vi "GetObjectFromMemory.vi"(8 "error in (no error)":errorcluster, 10 "ObjectName":string, 11 "Type":refnum<class>) -> (0 "error out":errorcluster, 3 "ObjectOut":refnum<class>)   [LabVIEW 2021, in "Application.lvclass"]
uses:
  Application.lvclass
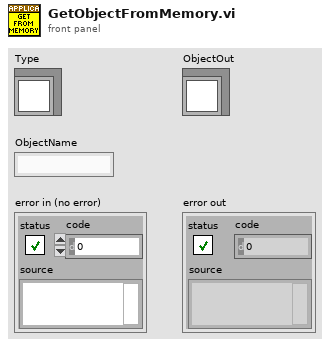
[diagram p1: front panel]
types:
  T1 = typedef "Application.lvclass/ObjectAttributes.ctl" = cluster{"Objects":variant, "BasePath":path, "Application":refnum<class "Application.lvclass">}
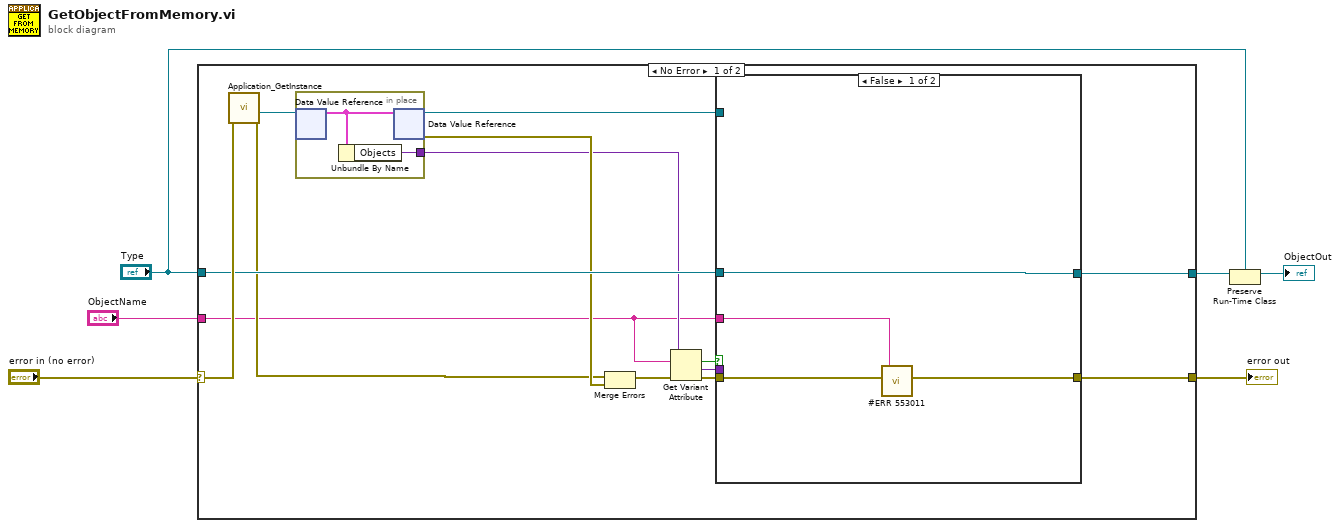
[diagram p0: block diagram]
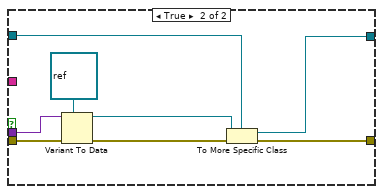
[diagram p2: hidden frame]
diagram:
  n1 = case shown="No Error" "error in (no error)" {
    selector: "error in (no error)" -> [w20 w35]
    tunnel: [w9 w35] -> w1
    tunnel: "ObjectName" -> [w7 _]
    tunnel: "Type" -> [w19 _]
    tunnel: [w18 _] -> w5
    frame No Error {
      n2 = call "Application_GetInstance.vi"("error in"=w20) -> ("error out"=w8:errorcluster, "DVRRefOut"=w16:refnum<data-value>)  [unwired: 6 in, 3 out]
      n3 = in-place {
        in-place-border: [w33] -> w11
        n4 = in-place-dvr #1(w16) -> (w34:T1)  [unwired: 1 out]
        n5 = Unbundle By Name(w34) -> ("Objects"=w33:variant)
        n6 = in-place-dvr #1(w34) -> (w10:refnum<data-value>, w17:errorcluster)
      }
      n7 = Merge Errors(w8, w17) -> (w15:errorcluster)
      n8 = Get Variant Attribute(Variant=w11, name=w7, error in=w15) -> (found=w13:bool, value=w12:variant, error out=w14:errorcluster)  [unwired: 1 in, 1 out]
      n9 = case shown="False" w13 {
        tunnel: w14 -> [w23 w32]
        tunnel: w19 -> [w24 w28]
        tunnel: [w22 w30] -> w9
        tunnel: [w24 w26] -> w18
        tunnel: w7 -> [w21 _]
        tunnel: w12 -> [_ w25]
        tunnel: w10 -> [_ _]
        frame False {
          n10 = call "#ERR 553011"("Data"=w21, "error in (no error)"=w23) -> ("error out"=w22:errorcluster)  [unwired: 9 in]
        }
        frame True {
          n11 = Variant To Data(error in=w32, type=refnum<class> refnum ("Type"), Variant=w25) -> (data=w27:refnum<class>, error out=w31:errorcluster)
          n12 = To More Specific Class(target class=w28, reference=w27, error in=w31) -> (specific class reference=w26:refnum<class>, error out=w30:errorcluster)
        }
      }
    }
    frame Error {
    }
  }
  "error out" <- w1
  n13 = Preserve Run-Time Class(object in=w5, 2:"Type") -> (object out=→"ObjectOut":refnum<class>)  [unwired: 1 in, 1 out]
